vi "Set value AR.vi"(7 "Ignore range overflow error (false)":bool, 8 "error in":errorcluster, 9 "Voltage frequnecy limit (none)":T1(ring), 10 "Value":dbl, 11 "VISA resource name":refnum<visa-resource-name>) -> (0 "error out":errorcluster, 2 "Set value failed":bool, 3 "VISA resource name out":refnum<visa-resource-name>)   [LabVIEW 2020, in "Datron D4xxx.lvlib"]
doc: "This VI sets main register value. Compared to \"Set value\" VI it don't just changes value of main register but it also sets corresponding range for it (autorange without R0 range selected). \nOptionally it can be configured to ignore error code returned by instrument after range/value/frequency command."
uses:
  Datron D4xxx.lvlib
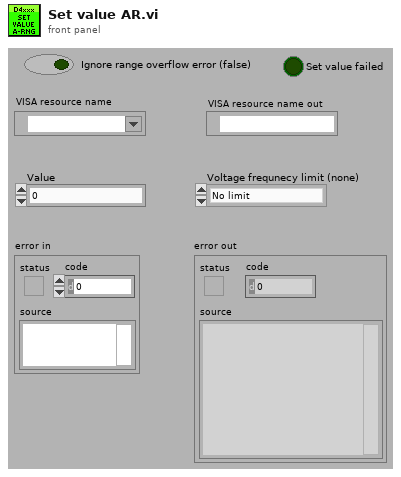
[diagram p1: front panel]
types:
  T1 = enum16{"No limit", "Always to 1kHz", "D4800", "D4805", "D4808"}
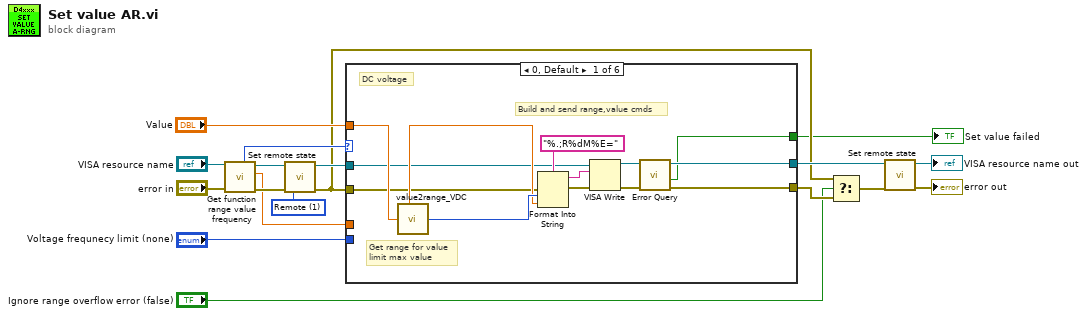
[diagram p0: block diagram]
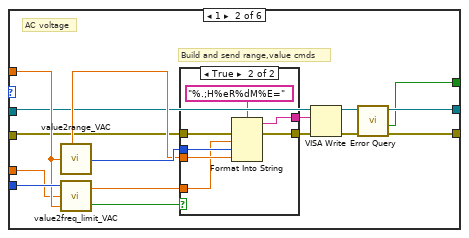
[diagram p2: hidden frame]
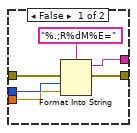
[diagram p3: hidden frame]
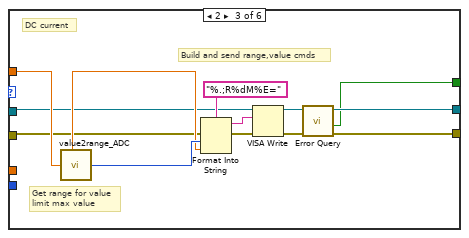
[diagram p4: hidden frame]
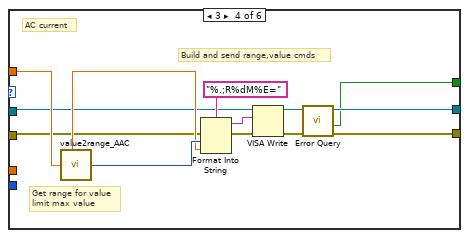
[diagram p5: hidden frame]
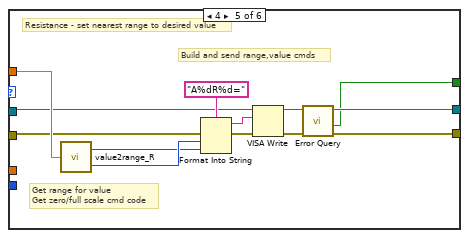
[diagram p6: hidden frame]
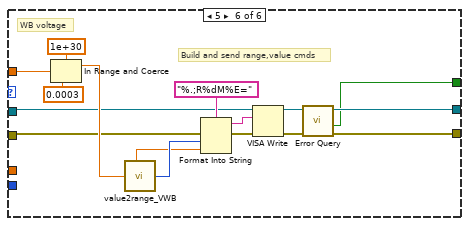
[diagram p7: hidden frame]
diagram:
  w13 = u16 1 items=["Local", "Remote", "Default"] ("Remote state")
  n1 = call "Get function range value frequency.vi"("error in (no error)"="error in", "VISA resource name"="VISA resource name") -> ("error out"=w12:errorcluster, "Frequency [Hz]"=w9:dbl, "VISA resource name out"=w11:refnum<visa-resource-name>, "Fucntion code"=w15:i32)  [unwired: 2 in, 4 out]
  n2 = call "Set remote state.vi"("error in"=w12, "Remote state"=w13, "VISA resource name"=w11) -> ("error out"=w3:errorcluster, "VISA resource name out"=w10:refnum<visa-resource-name>)  [unwired: 7 in]
  n3 = case shown="0, Default" w15 {
    tunnel: "Value" -> [w30 w40 w72 w85 w99 w110]
    tunnel: [w21 w34 w62 w76 w89 w102] -> w4
    tunnel: [w20 w33 w63 w75 w88 w101] -> w7
    tunnel: "Voltage frequnecy limit (none)" -> [_ w41 _ _ _ _]
    tunnel: w3 -> [w23 w35 w64 w78 w90 w103]
    tunnel: w10 -> [w22 w36 w65 w77 w91 w104]
    tunnel: w9 -> [_ w37 _ _ _ _]
    tunnel: [w19 w32 w61 w74 w87 w100] -> w1
    frame 0, Default {
      # "Build and send range,value cmds"
      # "Get range for value\nlimit max value"
      # "DC voltage"
      n4 = call "value2range_VDC.vi"("Voltage [V]"=w30) -> ("Limited voltage [V]"=w29:dbl, "Range [-]"=w31:i32)  [unwired: 1 in, 6 out]
      n5 = Format Into String(format string="%.;R%dM%E=", error in=w23, w31, w29) -> (resulting string=w28:string, error out=w27:errorcluster)  [unwired: 1 in]
      n6 = VISA Write(VISA resource name=w22, write buffer=w28, error in (no error)=w27) -> (VISA resource name out=w24:refnum<visa-resource-name>, error out=w25:errorcluster)  [unwired: 1 out]
      n7 = call "Error Query.vi"("error in (no error)"=w25, "VISA resource name"=w24) -> ("error out"=w21:errorcluster, "Error"=w19:bool, "VISA resource name out"=w20:refnum<visa-resource-name>)  [unwired: 6 in, 1 out]
    }
    frame 1 {
      # "Build and send range,value cmds"
      # "AC voltage"
      n8 = call "value2range_VAC.vi"("Voltage [V]"=w40) -> ("Limited voltage [V]"=w46:dbl, "Range [-]"=w47:i32)  [unwired: 3 in, 4 out]
      n9 = call "value2freq_limit_VAC.vi"("Voltage [V]"=w40, "Frequnecy [Hz]"=w37, "Limit type (none)"=w41) -> ("Limitation necessary"=w39:bool, "Limited frequency [V]"=w38:dbl)
      n10 = case shown="True" w39 {
        tunnel: w47 -> [w53 w60]
        tunnel: w46 -> [w52 w59]
        tunnel: [w51 w58] -> w45
        tunnel: [w50 w57] -> w44
        tunnel: w35 -> [w48 w55]
        tunnel: w38 -> [_ w54]
        frame False {
          n11 = Format Into String(format string="%.;R%dM%E=", error in=w48, w53, w52) -> (resulting string=w51:string, error out=w50:errorcluster)  [unwired: 1 in]
        }
        frame True {
          n12 = Format Into String(format string="%.;H%eR%dM%E=", error in=w55, w54, w60, w59) -> (resulting string=w58:string, error out=w57:errorcluster)  [unwired: 1 in]
        }
      }
      n13 = VISA Write(VISA resource name=w36, write buffer=w45, error in (no error)=w44) -> (VISA resource name out=w42:refnum<visa-resource-name>, error out=w43:errorcluster)  [unwired: 1 out]
      n14 = call "Error Query.vi"("error in (no error)"=w43, "VISA resource name"=w42) -> ("error out"=w34:errorcluster, "Error"=w32:bool, "VISA resource name out"=w33:refnum<visa-resource-name>)  [unwired: 6 in, 1 out]
    }
    frame 2 {
      # "Build and send range,value cmds"
      # "Get range for value\nlimit max value"
      # "DC current"
      n15 = call "value2range_ADC.vi"("Current [A]"=w72) -> ("Limited current [A]"=w71:dbl, "Range [-]"=w73:i32)  [unwired: 1 in, 6 out]
      n16 = Format Into String(format string="%.;R%dM%E=", error in=w64, w73, w71) -> (resulting string=w70:string, error out=w69:errorcluster)  [unwired: 1 in]
      n17 = VISA Write(VISA resource name=w65, write buffer=w70, error in (no error)=w69) -> (VISA resource name out=w66:refnum<visa-resource-name>, error out=w67:errorcluster)  [unwired: 1 out]
      n18 = call "Error Query.vi"("error in (no error)"=w67, "VISA resource name"=w66) -> ("error out"=w62:errorcluster, "Error"=w61:bool, "VISA resource name out"=w63:refnum<visa-resource-name>)  [unwired: 6 in, 1 out]
    }
    frame 3 {
      # "Build and send range,value cmds"
      # "Get range for value\nlimit max value"
      # "AC current"
      n19 = call "value2range_AAC.vi"("Current [A]"=w85) -> ("Limited current [A]"=w84:dbl, "Range [-]"=w86:i32)  [unwired: 3 in, 4 out]
      n20 = Format Into String(format string="%.;R%dM%E=", error in=w78, w86, w84) -> (resulting string=w83:string, error out=w82:errorcluster)  [unwired: 1 in]
      n21 = VISA Write(VISA resource name=w77, write buffer=w83, error in (no error)=w82) -> (VISA resource name out=w79:refnum<visa-resource-name>, error out=w80:errorcluster)  [unwired: 1 out]
      n22 = call "Error Query.vi"("error in (no error)"=w80, "VISA resource name"=w79) -> ("error out"=w76:errorcluster, "Error"=w74:bool, "VISA resource name out"=w75:refnum<visa-resource-name>)  [unwired: 6 in, 1 out]
    }
    frame 4 {
      # "Build and send range,value cmds"
      # "Get range for value\nGet zero/full scale cmd code"
      # "Resistance - set nearest range to desired value"
      n23 = call "value2range_R.vi"("Resistance [Ohm]"=w99) -> ("Nearest range code"=w92:i32, "Zero/full range code"=w93:i32)
      n24 = Format Into String(format string="A%dR%d=", error in=w90, w93, w92) -> (resulting string=w98:string, error out=w97:errorcluster)  [unwired: 1 in]
      n25 = VISA Write(VISA resource name=w91, write buffer=w98, error in (no error)=w97) -> (VISA resource name out=w94:refnum<visa-resource-name>, error out=w95:errorcluster)  [unwired: 1 out]
      n26 = call "Error Query.vi"("error in (no error)"=w95, "VISA resource name"=w94) -> ("error out"=w89:errorcluster, "Error"=w87:bool, "VISA resource name out"=w88:refnum<visa-resource-name>)  [unwired: 6 in, 1 out]
    }
    frame 5 {
      # "Build and send range,value cmds"
      # "WB voltage"
      n27 = In Range and Coerce(upper limit=1e+30, x=w110, lower limit=0.0003) -> (coerced(x)=w107:dbl)  [unwired: 1 out]
      n28 = call "value2range_VWB.vi"("Voltage [V]"=w107) -> ("Limited voltage [V]"=w105:dbl, "Range [-]"=w106:i32)  [unwired: 3 in, 4 out]
      n29 = Format Into String(format string="%.;R%dM%E=", error in=w103, w106, w105) -> (resulting string=w115:string, error out=w114:errorcluster)  [unwired: 1 in]
      n30 = VISA Write(VISA resource name=w104, write buffer=w115, error in (no error)=w114) -> (VISA resource name out=w111:refnum<visa-resource-name>, error out=w112:errorcluster)  [unwired: 1 out]
      n31 = call "Error Query.vi"("error in (no error)"=w112, "VISA resource name"=w111) -> ("error out"=w102:errorcluster, "Error"=w100:bool, "VISA resource name out"=w101:refnum<visa-resource-name>)  [unwired: 6 in, 1 out]
    }
  }
  "Set value failed" <- w1
  n32 = Select(t=w3, s="Ignore range overflow error (false)", f=w4) -> (s? t:f=w5:errorcluster)
  n33 = call "Set remote state.vi"("error in"=w5, "VISA resource name"=w7) -> ("error out"=→"error out":errorcluster, "VISA resource name out"=→"VISA resource name out":refnum<visa-resource-name>)  [unwired: 8 in]
